vi "New Observing ViewModel.vi"() -> (1 "Test Reply Queue":refnum<queue>, 3 "ObservingViewModel Out":refnum<class "ObservingViewModel.lvclass">)   [LabVIEW 2017, in "ObservingViewModel.lvclass"]
uses:
  ObservingViewModel.lvclass
  ObservingViewModel.lvclass/ObservingViewModel.ctl
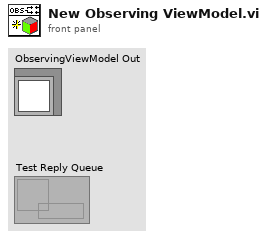
[diagram p1: front panel]
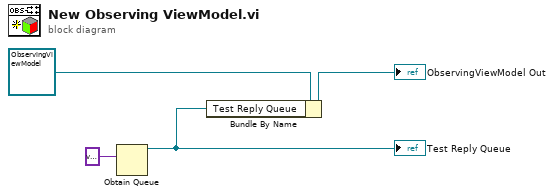
[diagram p0: block diagram]
diagram:
  n1 = Obtain Queue(element data type=variant) -> (queue out=w1:refnum<queue>)  [unwired: 4 in, 2 out]
  "Test Reply Queue" <- w1
  n2 = Bundle By Name(cluster=refnum<class "ObservingViewModel.lvclass"> refnum ("ObservingViewable in"), "Test Reply Queue"=w1) -> (→"ObservingViewModel Out":refnum<class "ObservingViewModel.lvclass">)
